vi "7.1 Manual Act Loop.vi"() -> ()   [LabVIEW 2010]
uses:
  4-High Neurons/4.0-Timing Badass.ctl
  6-OCU Neurons/6.1-Act.ctl
  6-OCU Neurons/6.1-UDP Saitek.ctl
  <vilib>/Utility/inputDevices.llb/closeJoystick.vi
  7.0-Global.vi
  <vilib>/Utility/inputDevices.llb/joystickAcquire.vi
panel:
  in  "Stop":bool
  out "output cluster":T1 {"6.1-Saitek Controller"."Right" scale=0.0..1.0; "6.1-Saitek Controller"."Left" scale=0.0..1.0; "6.1-Saitek Controller"."Yaw" scale=-1.0..1.0; "6.1-Saitek Controller"."Roll" scale=-1.0..1.0; "6.1-Saitek Controller"."Pitch" scale=-1.0..1.0}
  out "Super Heart Beat":T3
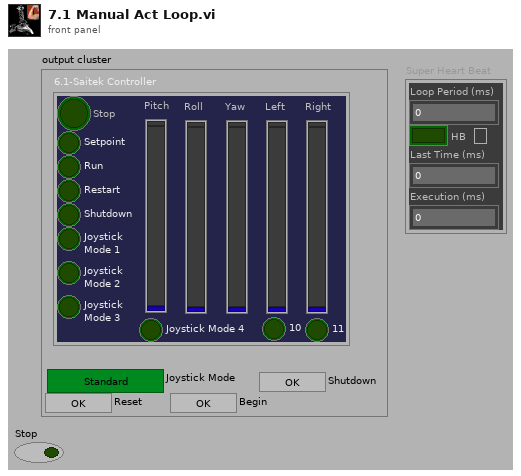
[diagram p1: front panel]
types:
  T1 = typedef "6.1-Act.ctl" = cluster{"6.1-Saitek Controller":T2, "Joystick Mode":bool, "Shutdown":bool, "Reset":bool, "Begin":bool}
  T2 = typedef "6.1-UDP Saitek.ctl" = cluster{"Stop":bool, "Setpoint":bool, "Run":bool, "Restart":bool, "Shutdown":bool, "Joystick\nMode 1":bool, "Joystick\nMode 2":bool, "Joystick \nMode 3":bool, "Joystick Mode 4":bool, "10":bool, "11":bool, "Pitch":sgl, "Roll":sgl, "Yaw":sgl, "Left":sgl, "Right":sgl}
  T3 = typedef "4.0-Timing Badass.ctl" = cluster{"Loop Period (ms)":u32, "HB":bool, "Last Time (ms)":u32, "Execution (ms)":u32}
  T4 = typedef "7.0 Manual Mode Buttons.ctl" = cluster{"Joystick Mode":bool, "Reset":bool, "Begin":bool}
  T5 = cluster{"X axis":i32, "Y axis":i32, "Z axis":i32, "X axis rotation":i32, "Y axis rotation":i32, "Z axis rotation":i32, "U axis":i32, "V axis":i32}
  T6 = cluster{"button 1":bool, "button 2":bool, "button 3":bool, "button 4":bool, "button 5":bool, "button 6":bool, "button 7":bool, "button 8":bool, "button 9":bool, "button 10":bool, "button 11":bool, "button 12":bool, "button 13":bool, "button 14":bool, "button 15":bool, "button 16":bool, "button 17":bool, "button 18":bool, "button 19":bool, "button 20":bool, "button 21":bool, "button 22":bool, "button 23":bool, "button 24":bool, "button 25":bool, "button 26":bool, "button 27":bool, "button 28":bool, "button 29":bool, "button 30":bool, "button 31":bool, "button 32":bool}
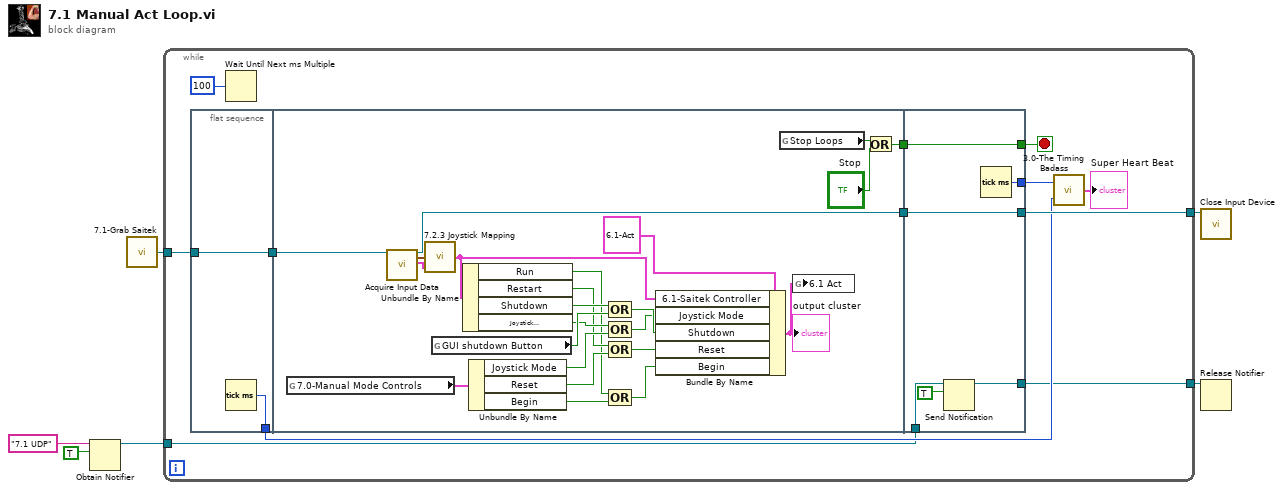
[diagram p0: block diagram]
diagram:
  n1 = Obtain Notifier(name (unnamed)="7.1 UDP", notification data type=TRUE) -> (notifier out=w2:refnum<notifier>)  [unwired: 2 in, 2 out]
  n2 = call "7.1-Grab Saitek.vi"() -> ("Saitek ID"=w5:refnum<k1>)
  n3 = while {
    tunnel: w5 -> [w17]
    tunnel: [w16] -> w6
    tunnel: w2 -> [w8]
    tunnel: [w7] -> w1
    stop <- w18 stop-if-true
    n4 = flat-sequence {
      tunnel: w17 -> [w20]
      tunnel: [w20] -> w13
      tunnel: [w19] -> w11
      tunnel: [w33] -> w15
      tunnel: [w39] -> w14
      tunnel: w13 -> [w42]
      tunnel: [w48] -> w16
      tunnel: [w49] -> w18
      tunnel: w15 -> [w49]
      tunnel: w14 -> [w48]
      tunnel: [w47] -> w12
      tunnel: w8 -> [w46]
      tunnel: [w44] -> w7
      frame #0 {
        n5 = Tick Count (ms)() -> (millisecond timer value=w19:u32)
      }
      frame #1 {
        n6 = global read "7.0-Global.vi" "7.0-Manual Mode Controls"() -> (w36:T4)
        n7 = call-poly <vilib>:"Acquire Input Data.vi"("device ID"=w42) -> ("device ID"=w39:refnum<k1>, "axis info"=w41:T5, "button info"=w40:T6)  [unwired: 14 in, 2 out]
        n8 = call "7.2.3 Joystick Mapping.vi"("button info"=w40, "axis info"=w41) -> ("Joystick Out"=w31:T2)  [unwired: 1 in]
        n9 = global read "7.0-Global.vi" "GUI shutdown Button"() -> (w29:bool)
        n10 = Unbundle By Name(w31) -> ("Run"=w21:bool, "Restart"=w22:bool, "Shutdown"=w24:bool, "Joystick \nMode 3"=w23:bool)
        n11 = Unbundle By Name(w36) -> ("Joystick Mode"=w30:bool, "Reset"=w35:bool, "Begin"=w34:bool)
        n12 = Compound Arithmetic op=OR(w24, w29) -> (w28:bool)
        n13 = Compound Arithmetic op=OR(w23, w30) -> (w27:bool)
        n14 = Compound Arithmetic op=OR(w22, w35) -> (w26:bool)
        n15 = Compound Arithmetic op=OR(w21, w34) -> (w25:bool)
        n16 = Bundle By Name(cluster=T1 {"6.1-Saitek Controller"={"Stop"=FALSE, "Setpoint"=FALSE, "Run"=FALSE, "Restart"=FALSE, "Shutdown"=FALSE, "Joystick\nMode 1"=FALSE, "Joystick\nMode 2"=FALSE, "Joystick \nMode 3"=FALSE, "Joystick Mode 4"=FALSE, "10"=FALSE, "11"=FALSE, "Pitch"=0.0, "Roll"=0.0, "Yaw"=0.0, "Left"=0.0, "Right"=0.0}, "Joystick Mode"=FALSE, "Shutdown"=FALSE, "Reset"=FALSE, "Begin"=FALSE} ("6.1 Act"), "6.1-Saitek Controller"=w31, "Joystick Mode"=w27, "Shutdown"=w28, "Reset"=w26, "Begin"=w25) -> (w37:T1)
        "output cluster" <- w37
        n17 = global read "7.0-Global.vi" "Stop Loops"() -> (w43:bool)
        n18 = global write "7.0-Global.vi" "6.1 Act"(w37) -> ()
        n19 = Or(x=w43, y="Stop") -> (x .or. y?=w33:bool)
      }
      frame #2 {
        n20 = Send Notification(notification=TRUE, notifier=w46) -> (notifier out=w44:refnum<notifier>)  [unwired: 1 in, 1 out]
        n21 = Tick Count (ms)() -> (millisecond timer value=w47:u32)
      }
    }
    n22 = Wait Until Next ms Multiple(millisecond multiple=u32 100) -> ()  [unwired: 1 out]
    n23 = call "3.0-The Timing Badass.vi"("Start"=w11, "End"=w12) -> ("Super Heart Beat"=→"Super Heart Beat":T3)
  }
  n24 = call-poly <vilib>:"Close Input Device.vi"("device ID"=w6) -> ()  [unwired: 9 in, 1 out]
  n25 = Release Notifier(notifier=w1) -> ()  [unwired: 2 in, 3 out]
